vi "Agilent VNA Sort Measurements.vi"(7 "Agilent VNA":T6, 8 "error in (no error)":errorcluster, 9 "Auto Select":bool, 10 "Parameters to Measure":T1[](array[typedef]) {"Channel" min=1 max=99 step=1; "Parameter"."Stimulus Port" min=1 step=1; "Parameter"."Response Port" min=1 step=1}, 11 "VISA Resource Name":refnum<visa-resource-name>) -> (0 "error out":errorcluster {"code" format="%.0x"}, 1 "Channels Used":i8[](array[numeric]), 2 "Sorted Measurements":cluster{"Measurements":T5[]}[](array[cluster]) {"Measurements"."Traces"."Parameter"."Stimulus Port" min=1 step=1; "Measurements"."Traces"."Parameter"."Response Port" min=1 step=1}, 3 "dup VISA Resource Name":refnum<visa-resource-name>, 4 "Sorted Parameters to Measure":T1[](array[typedef]) {"Channel" min=1 max=99 step=1; "Parameter"."Stimulus Port" min=1 step=1; "Parameter"."Response Port" min=1 step=1}, 5 "Removed Parameters":T1[](array[typedef]) {"Channel" min=1 max=99 step=1; "Parameter"."Stimulus Port" min=1 step=1; "Parameter"."Response Port" min=1 step=1}, 6 "Measurements Removed?":bool)   [LabVIEW 2011]
uses:
  tests/S Parameter/TypeDefs/SP Parameter to Measure.ctl
  tests/S Parameter/TypeDefs/SP Parameter.ctl
  tests/S Parameter/TypeDefs/SP Calibration State.ctl
  tests/S Parameter/TypeDefs/SP Measurement Format.ctl
  TypeDefs/Agilent VNA Instrument Info.ctl
  TypeDefs/Agilent VNA Measurements.ctl
  SI.LIB/Add to Array if Not Present (I32).vi
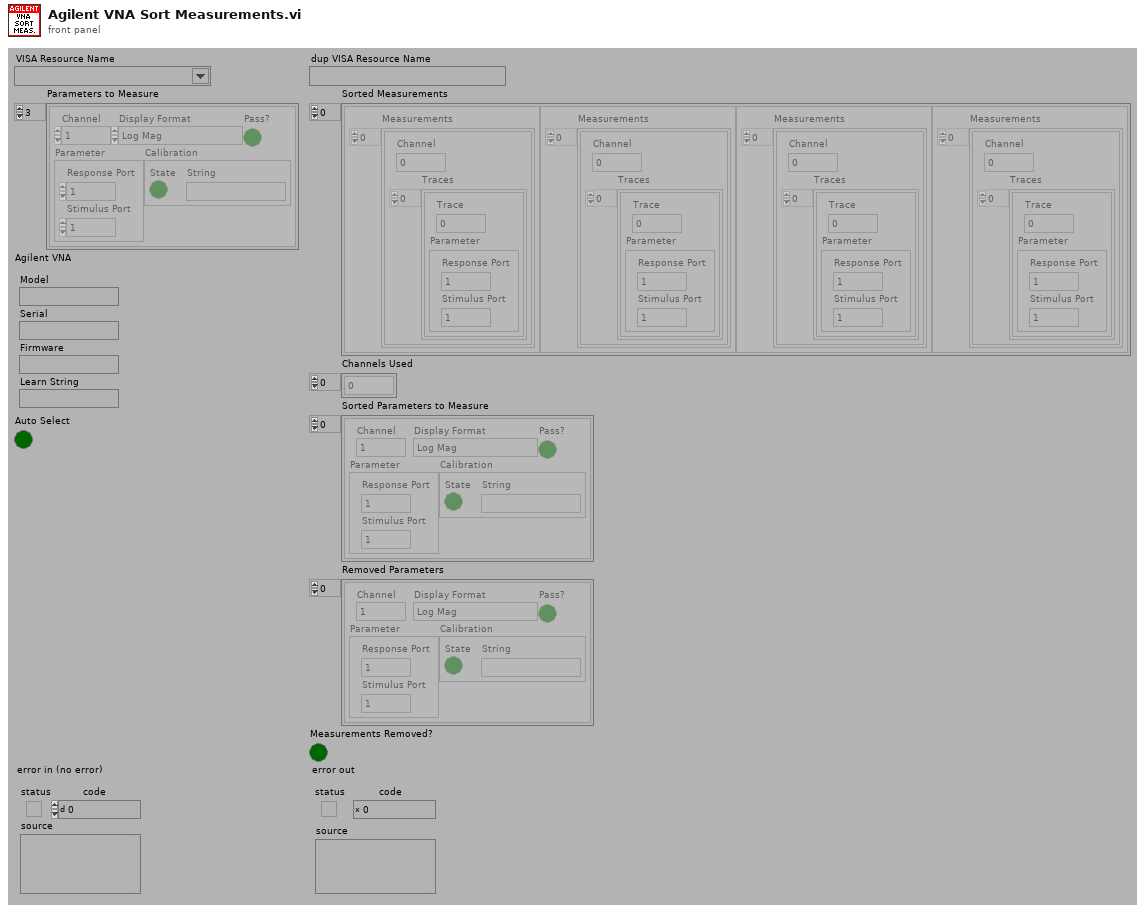
[diagram p1: front panel]
types:
  T1 = typedef "SP Parameter to Measure.ctl" = cluster{"Channel":i8, "Parameter":T2, "Calibration":T3, "Display Format":T4, "Pass?":bool}
  T2 = typedef "SP Parameter.ctl" = cluster{"Stimulus Port":i8, "Response Port":i8}
  T3 = typedef "SP Calibration State.ctl" = cluster{"State":bool, "String":string}
  T4 = typedef "SP Measurement Format.ctl" = enum32{"Log Mag", "Phase", "Delay", "Smith (R+jX)", "Polar (Re/Im)", "Linear Mag", "SWR", "Real", "Imaginary", "Smith (Lin/Phase)", "Smith (Log/Phase)", "Smith (Real/Imag)", "Smith (G+jB)", "Polar (Lin/Phase)", "Polar (Log/Phase)", "Expanded Phase", "Positive Phase", "Inverted Smith", "Unwrapped Phase", "Power Out", "Power In", "Linear Mag/Phase", "Log Mag/Phase", "Real/Imaginary"}
  T5 = typedef "Agilent VNA Measurements.ctl" = cluster{"Channel":i8, "Traces":cluster{"Trace":i8, "Parameter":T2}[]}
  T6 = typedef "Agilent VNA Instrument Info.ctl" = cluster{"Model":string, "Serial":string, "Firmware":string, "Learn String":string}
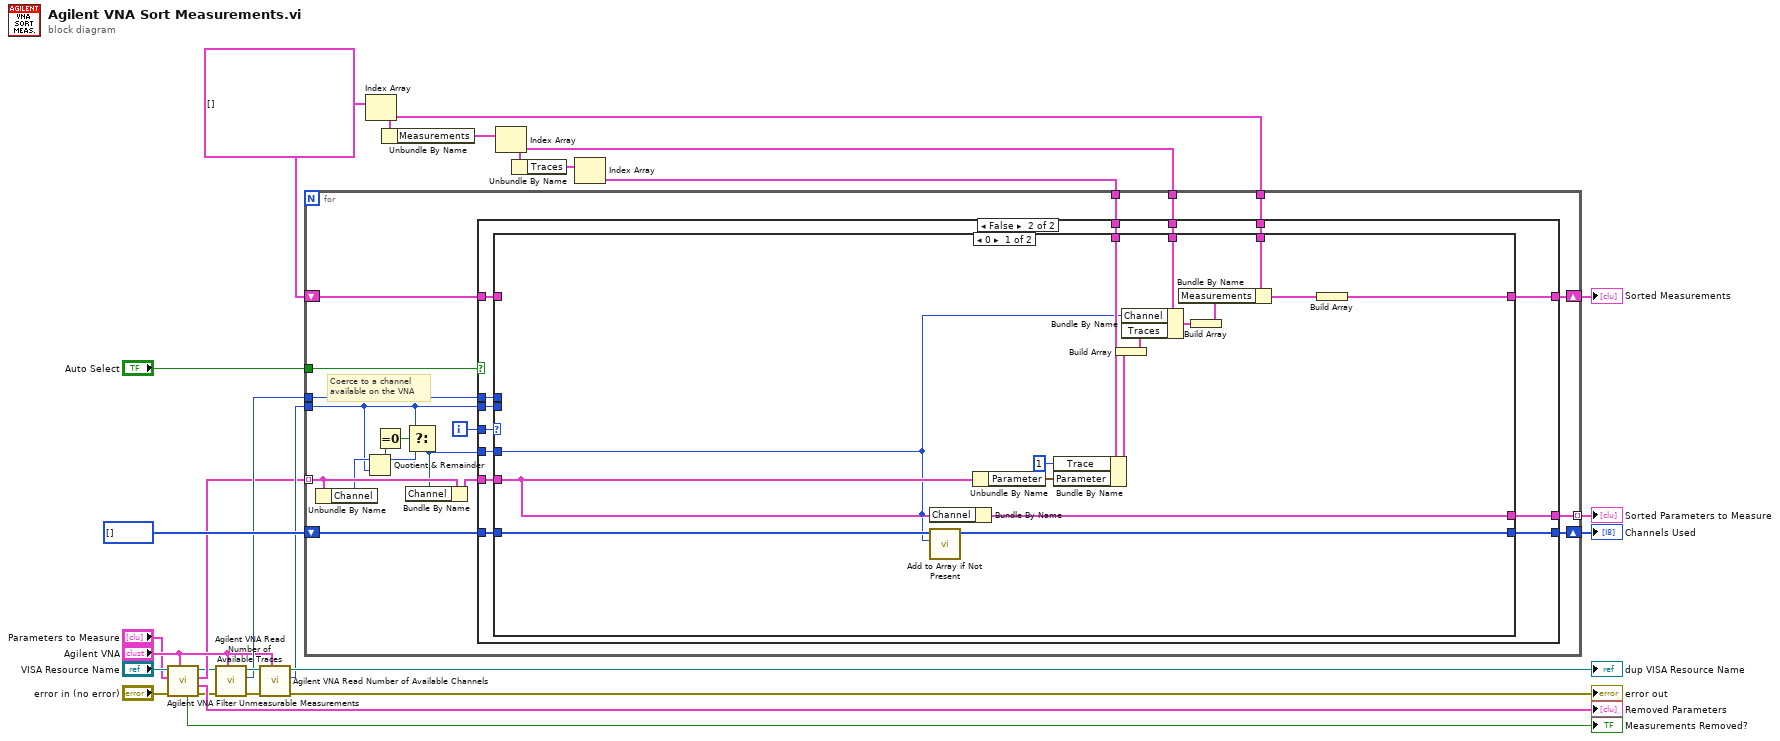
[diagram p0: block diagram]
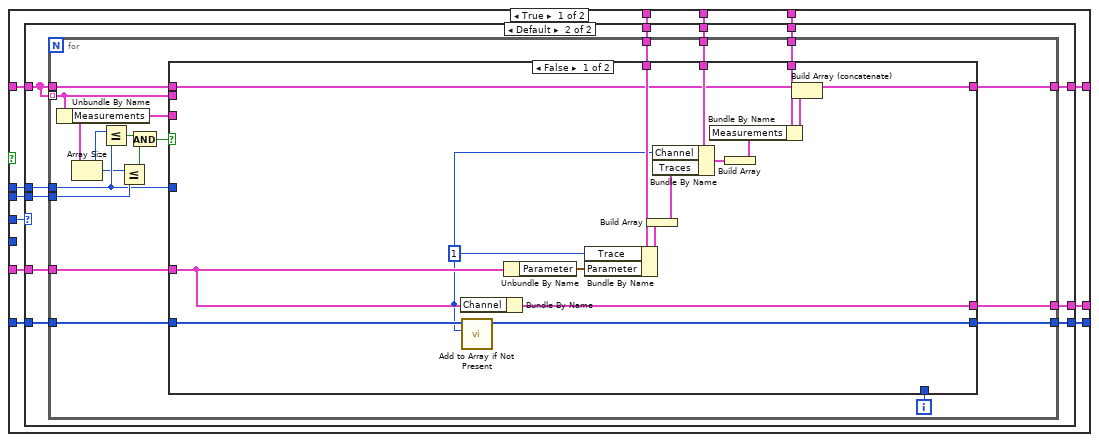
[diagram p2: hidden frame]
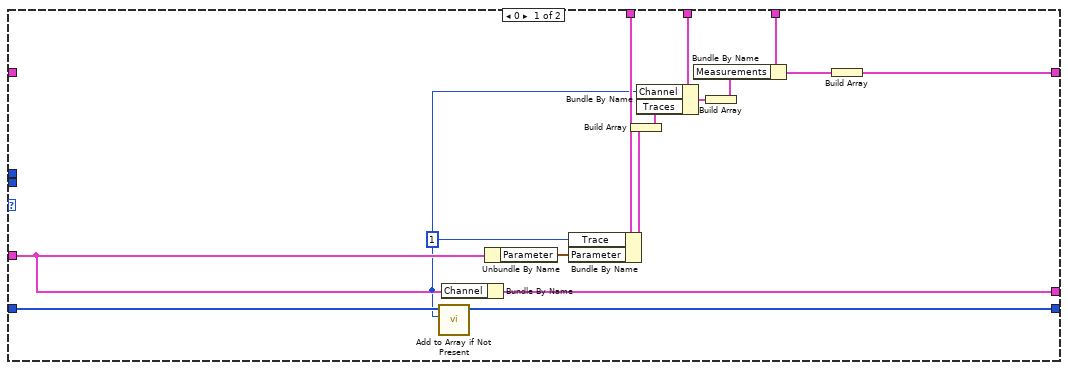
[diagram p3: hidden frame]
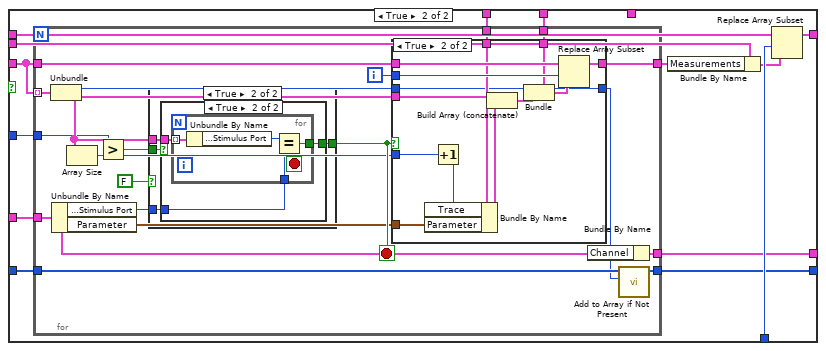
[diagram p4: hidden frame]
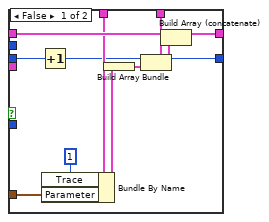
[diagram p7: hidden frame]
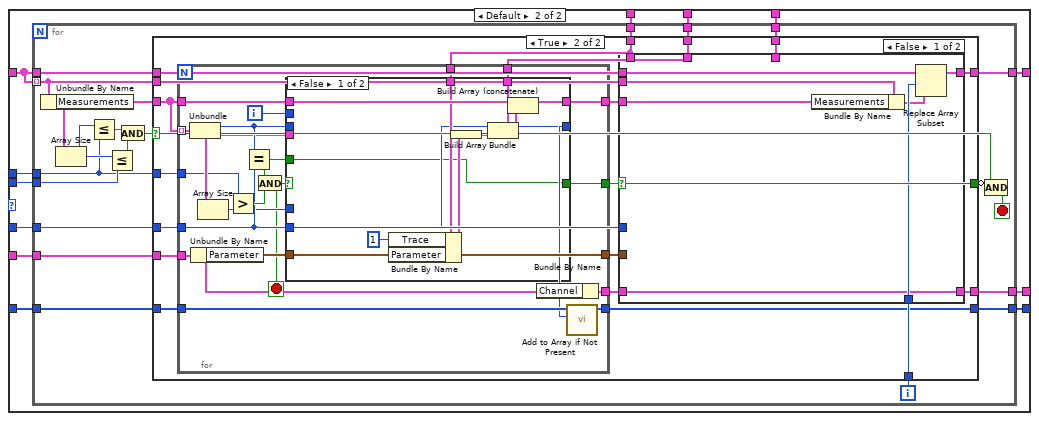
[diagram p8: hidden frame]
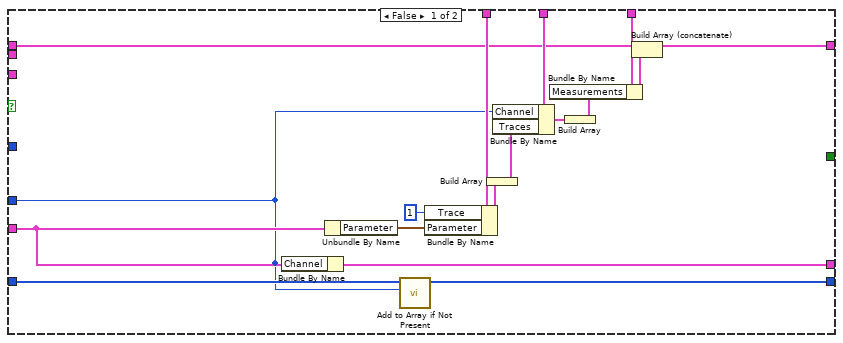
[diagram p9: hidden frame]
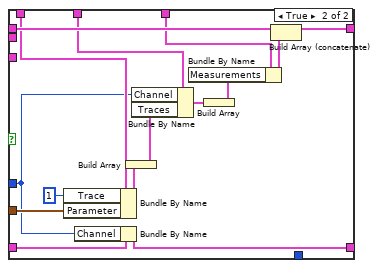
[diagram p10: hidden frame]
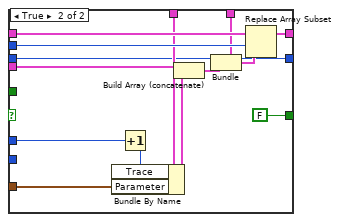
[diagram p11: hidden frame]
diagram:
  w21 = cluster{"Measurements":T5[]}[] [] ("Sorted Measurements")
  n1 = call "Agilent VNA Filter Unmeasurable Measurements.vi"("Agilent VNA"="Agilent VNA", "error in (no error)"="error in (no error)", "Parameters to Measure"="Parameters to Measure", "VISA Resource Name"="VISA Resource Name") -> ("error out"=w1:errorcluster, "Removed Parameters"=→"Removed Parameters":T1[], "Filtered Parameters to Measure"=w6:T1[], "dup VISA Resource Name"=w2:refnum<visa-resource-name>, "Measurements Removed?"=→"Measurements Removed?":bool)  [unwired: 3 out]
  n2 = call "Agilent VNA Read Number of Available Traces.vi"("Agilent VNA"="Agilent VNA", "error in (no error)"=w1, "VISA Resource Name"=w2) -> ("error out"=w13:errorcluster, "Number of Traces"=w11:i8, "dup VISA Resource Name"=w12:refnum<visa-resource-name>)  [unwired: 6 out]
  n3 = call "Agilent VNA Read Number of Available Channels.vi"("Agilent VNA"="Agilent VNA", "error in (no error)"=w13, "VISA Resource Name"=w12) -> ("error out"=→"error out":errorcluster, "Number of Channels"=w14:i8, "dup VISA Resource Name"=→"dup VISA Resource Name":refnum<visa-resource-name>)  [unwired: 6 out]
  n4 = Index Array(array=w21) -> (element=w17:cluster{"Measurements":T5[]})  [unwired: 1 in]
  n5 = Unbundle By Name(w17) -> ("Measurements"=w23:T5[])
  n6 = Index Array(array=w23) -> (element=w18:T5)  [unwired: 1 in]
  n7 = Unbundle By Name(w18) -> ("Traces"=w20:cluster{"Trace":i8, "Parameter":T2}[])
  n8 = Index Array(array=w20) -> (element=w19:cluster{"Trace":i8, "Parameter":T2})  [unwired: 1 in]
  n9 = for {
    tunnel: w6 -> [w42] mode=indexing
    shift-right: [w32] -> w22
    shift-left: w21 -> [w43]
    tunnel: w14 -> [w37]
    tunnel: "Auto Select" -> [w35]
    tunnel: w19 -> [w34]
    tunnel: w18 -> [w33]
    tunnel: w17 -> [w31]
    shift-right: [w29] -> w15
    shift-left: i8[] [] -> [w30]
    tunnel: w11 -> [w28]
    tunnel: [w27] -> w5 mode=indexing
    i -> [w44]
    # "Coerce to a channel\navailable on the VNA"
    n10 = Unbundle By Name(w42) -> ("Channel"=w40:i8)
    n11 = Quotient & Remainder(x=w40, y=w37) -> (x-y*floor(x/y)=w36:i8)  [unwired: 1 out]
    n12 = Equal To 0?(x=w36) -> (x = 0?=w39:bool)
    n13 = Select(t=w37, s=w39, f=w36) -> (s? t:f=w38:i8)
    n14 = Bundle By Name(cluster=w42, "Channel"=w38) -> (w41:T1)
    n15 = case shown="False" w35 {
      tunnel: w44 -> [w50 w194]
      tunnel: w43 -> [w56 w200]
      tunnel: w41 -> [w55 w199]
      tunnel: w38 -> [_ w190]
      tunnel: w37 -> [w54 w198]
      tunnel: w34 -> [w53 w197]
      tunnel: w33 -> [w52 w196]
      tunnel: [w51 w195] -> w32
      tunnel: w31 -> [w49 w193]
      tunnel: w30 -> [w48 w192]
      tunnel: [w47 w191] -> w29
      tunnel: w28 -> [w46 w189]
      tunnel: [w45 w188] -> w27
      frame True {
        n16 = case shown="Default" w50 {
          tunnel: w56 -> [_ w77]
          tunnel: w55 -> [w59 w82]
          tunnel: w54 -> [_ w81]
          tunnel: w53 -> [w71 w80]
          tunnel: w52 -> [w69 w79]
          tunnel: [w62 w78] -> w51
          tunnel: w49 -> [w65 w76]
          tunnel: w48 -> [w61 w75]
          tunnel: [w60 w74] -> w47
          tunnel: w46 -> [_ w73]
          tunnel: [w57 w72] -> w45
          frame 0 {
            w58 = i8 1 ("Trace")
            n17 = call-poly "Add to Array if Not Present.vi"("I32"=w58, "I32 Array"=w61) -> ("New I32 Array"=w60:i32[])  [unwired: 3 out]
            n18 = Bundle By Name(cluster=w59, "Channel"=w58) -> (w57:T1)
            n19 = Unbundle By Name(w59) -> ("Parameter"=w70:T2)
            n20 = Bundle By Name(cluster=w71, "Trace"=w58, "Parameter"=w70) -> (w67:cluster{"Trace":i8, "Parameter":T2})
            n21 = Build Array(w67) -> (w66:cluster{"Trace":i8, "Parameter":T2}[])
            n22 = Bundle By Name(cluster=w69, "Channel"=w58, "Traces"=w66) -> (w68:T5)
            n23 = Build Array(w68) -> (w64:T5[])
            n24 = Bundle By Name(cluster=w65, "Measurements"=w64) -> (w63:cluster{"Measurements":T5[]})
            n25 = Build Array(w63) -> (w62:cluster{"Measurements":T5[]}[])
          }
          frame Default {
            n26 = for {
              tunnel: w77 -> [w96]
              tunnel: w82 -> [w100]
              tunnel: w81 -> [w85]
              tunnel: w80 -> [w99]
              tunnel: w79 -> [w98]
              tunnel: [w97] -> w78
              tunnel: w77 -> [w92] mode=indexing
              tunnel: w76 -> [w93]
              tunnel: w75 -> [w91]
              tunnel: [w90] -> w74
              tunnel: w73 -> [w84]
              tunnel: [w89] -> w72
              i -> [w95]
              n27 = Unbundle By Name(w92) -> ("Measurements"=w94:T5[])
              n28 = Array Size(array=w94) -> (size(s)=w83:i32)
              n29 = Less Or Equal?(x=w83, y=w84) -> (x <= y?=w87:bool)
              n30 = Less Or Equal?(x=w83, y=w85) -> (x <= y?=w88:bool)
              n31 = And(x=w87, y=w88) -> (x .and. y?=w86:bool)
              n32 = case shown="False" w86 {
                tunnel: w100 -> [w103 w130]
                tunnel: w99 -> [w114 w129]
                tunnel: w98 -> [w113 w128]
                tunnel: [w116 w125] -> w97
                tunnel: w94 -> [_ w127]
                tunnel: w96 -> [w110 w126]
                tunnel: w95 -> [_ w124]
                tunnel: w93 -> [w108 _]
                tunnel: w92 -> [_ w123]
                tunnel: w91 -> [w105 w120]
                tunnel: [w104 w119] -> w90
                tunnel: w84 -> [_ w118]
                tunnel: [w102 w117] -> w89
                frame False {
                  w101 = i8 1 ("Channel")
                  n33 = Bundle By Name(cluster=w103, "Channel"=w101) -> (w102:T1)
                  n34 = call-poly "Add to Array if Not Present.vi"("I32"=w101, "I32 Array"=w105) -> ("New I32 Array"=w104:i32[])  [unwired: 3 out]
                  n35 = Unbundle By Name(w103) -> ("Parameter"=w115:T2)
                  n36 = Bundle By Name(cluster=w114, "Trace"=w101, "Parameter"=w115) -> (w112:cluster{"Trace":i8, "Parameter":T2})
                  n37 = Build Array(w112) -> (w111:cluster{"Trace":i8, "Parameter":T2}[])
                  n38 = Bundle By Name(cluster=w113, "Channel"=w101, "Traces"=w111) -> (w109:T5)
                  n39 = Build Array(w109) -> (w107:T5[])
                  n40 = Bundle By Name(cluster=w108, "Measurements"=w107) -> (w106:cluster{"Measurements":T5[]})
                  n41 = Build Array (concatenate)(w110, w106) -> (w116:cluster{"Measurements":T5[]}[])
                }
                frame True {
                  n42 = for {
                    tunnel: w127 -> [w146] mode=indexing
                    tunnel: w130 -> [w134]
                    tunnel: w127 -> [w150]
                    tunnel: [w147] -> w122
                    tunnel: w129 -> [w142]
                    tunnel: w128 -> [w140]
                    tunnel: w120 -> [w137]
                    tunnel: [w136] -> w119
                    tunnel: w118 -> [w135]
                    tunnel: [w133] -> w117
                    i -> [w149]
                    stop <- w145 stop-if-true
                    n43 = Unbundle(w146) -> ("Channel"=w143:i8, "Traces"=w144:cluster{"Trace":i8, "Parameter":T2}[])
                    n44 = Unbundle By Name(w134) -> ("Parameter.Stimulus Port"=w138:i8, "Parameter"=w139:T2)
                    n45 = Array Size(array=w144) -> (size(s)=w141:i32)
                    n46 = Greater?(x=w135, y=w141) -> (0:w148:bool)
                    n47 = case shown="True" FALSE {
                      tunnel: w148 -> [w151 w155]
                      tunnel: [w151 w154] -> w145
                      tunnel: w144 -> [_ w153]
                      tunnel: w138 -> [_ w152]
                      frame False {
                        # "We are no longer sorting by\nstimulus port.  We have decided\nthat it is no faster since it has to\nsweep once for each stimulus\nport no matter the configuration."
                      }
                      frame True {
                        n48 = case shown="True" w155 {
                          selector: w155 -> [w156 _]
                          tunnel: w153 -> [_ w159]
                          tunnel: [w156 w158] -> w154
                          tunnel: w152 -> [_ w157]
                          frame False {
                          }
                          frame True {
                            n49 = for {
                              tunnel: w159 -> [w163] mode=indexing
                              tunnel: [w161] -> w158
                              tunnel: w157 -> [w160]
                              stop <- w161 stop-if-true
                              n50 = Unbundle By Name(w163) -> ("Parameter.Stimulus Port"=w162:i8)
                              n51 = Equal?(x=w162, y=w160) -> (x = y?=w161:bool)
                            }
                          }
                        }
                      }
                    }
                    n52 = case shown="True" w145 {
                      tunnel: w144 -> [_ w183]
                      tunnel: w150 -> [w174 w187]
                      tunnel: w149 -> [_ w186]
                      tunnel: [w173 w185] -> w147
                      tunnel: w143 -> [w166 w175]
                      tunnel: w139 -> [w169 w181]
                      tunnel: w142 -> [w168 w182]
                      tunnel: w141 -> [_ w180]
                      tunnel: w140 -> [w170 w177]
                      tunnel: [w164 w175] -> w132
                      frame False {
                        n53 = Increment(x=w166) -> (x+1=w164:i8)
                        n54 = Bundle By Name(cluster=w168, "Trace"=i8 1, "Parameter"=w169) -> (w167:cluster{"Trace":i8, "Parameter":T2})
                        n55 = Build Array(w167) -> (w171:cluster{"Trace":i8, "Parameter":T2}[])
                        n56 = Bundle(cluster=w170, "Channel"=w164, "Traces"=w171) -> (w172:T5)
                        n57 = Build Array (concatenate)(w174, w172) -> (w173:T5[])
                      }
                      frame True {
                        n58 = Increment(x=w180) -> (x+1=w179:i32)
                        n59 = Bundle By Name(cluster=w182, "Trace"=w179, "Parameter"=w181) -> (w178:cluster{"Trace":i8, "Parameter":T2})
                        n60 = Build Array (concatenate)(w183, w178) -> (w176:cluster{"Trace":i8, "Parameter":T2}[])
                        n61 = Bundle(cluster=w177, "Channel"=w175, "Traces"=w176) -> (w184:T5)
                        n62 = Replace Array Subset(array=w187, new element=w184, index=w186) -> (w185:T5[])
                      }
                    }
                    n63 = Bundle By Name(cluster=w134, "Channel"=w132) -> (w133:T1)
                    n64 = call-poly "Add to Array if Not Present.vi"("I32"=w132, "I32 Array"=w137) -> ("New I32 Array"=w136:i32[])  [unwired: 3 out]
                  }
                  n65 = Bundle By Name(cluster=w123, "Measurements"=w122) -> (w121:cluster{"Measurements":T5[]})
                  n66 = Replace Array Subset(array=w126, new element=w121, index=w124) -> (w125:cluster{"Measurements":T5[]}[])
                }
              }
            }
          }
        }
      }
      frame False {
        n67 = case shown="0" w194 {
          tunnel: w200 -> [_ w223]
          tunnel: w199 -> [w204 w228]
          tunnel: w198 -> [_ w227]
          tunnel: w197 -> [w216 w226]
          tunnel: w196 -> [w214 w225]
          tunnel: [w207 w224] -> w195
          tunnel: w193 -> [w210 w222]
          tunnel: w192 -> [w206 w221]
          tunnel: [w205 w220] -> w191
          tunnel: w190 -> [w201 w219]
          tunnel: w189 -> [_ w218]
          tunnel: [w203 w217] -> w188
          frame 0 {
            n68 = Bundle By Name(cluster=w204, "Channel"=w201) -> (w203:T1)
            n69 = call-poly "Add to Array if Not Present.vi"("I32"=w201, "I32 Array"=w206) -> ("New I32 Array"=w205:i32[])  [unwired: 3 out]
            n70 = Unbundle By Name(w204) -> ("Parameter"=w215:T2)
            n71 = Bundle By Name(cluster=w216, "Trace"=i8 1 ("Channel"), "Parameter"=w215) -> (w212:cluster{"Trace":i8, "Parameter":T2})
            n72 = Build Array(w212) -> (w211:cluster{"Trace":i8, "Parameter":T2}[])
            n73 = Bundle By Name(cluster=w214, "Channel"=w201, "Traces"=w211) -> (w213:T5)
            n74 = Build Array(w213) -> (w209:T5[])
            n75 = Bundle By Name(cluster=w210, "Measurements"=w209) -> (w208:cluster{"Measurements":T5[]})
            n76 = Build Array(w208) -> (w207:cluster{"Measurements":T5[]}[])
          }
          frame Default {
            n77 = for {
              tunnel: w223 -> [w245]
              tunnel: w228 -> [w249]
              tunnel: w227 -> [w231]
              tunnel: w226 -> [w248]
              tunnel: w225 -> [w247]
              tunnel: [w246] -> w224
              tunnel: w223 -> [w242] mode=indexing
              tunnel: w222 -> [w243]
              tunnel: w221 -> [w241]
              tunnel: [w240] -> w220
              tunnel: w219 -> [w239]
              tunnel: w218 -> [w229]
              tunnel: [w236] -> w217
              i -> [w244]
              stop <- w237 stop-if-true
              n78 = Unbundle By Name(w242) -> ("Measurements"=w233:T5[])
              n79 = Array Size(array=w233) -> (size(s)=w230:i32)
              n80 = Less Or Equal?(x=w230, y=w229) -> (x <= y?=w234:bool)
              n81 = Less Or Equal?(x=w230, y=w231) -> (x <= y?=w235:bool)
              n82 = And(x=w234, y=w235) -> (x .and. y?=w232:bool)
              n83 = case shown="True" w232 {
                tunnel: w249 -> [w252 w284]
                tunnel: w248 -> [w264 w275]
                tunnel: w247 -> [w263 w274]
                tunnel: [w266 w281] -> w246
                tunnel: w233 -> [_ w283]
                tunnel: w245 -> [w260 w282]
                tunnel: w244 -> [_ w280]
                tunnel: w243 -> [w258 w271]
                tunnel: w242 -> [_ w279]
                tunnel: w241 -> [w255 w277]
                tunnel: [w254 w276] -> w240
                tunnel: w239 -> [w251 w272]
                tunnel: [_ w270] -> w238
                tunnel: w229 -> [_ w269]
                tunnel: [w250 w268] -> w236
                frame False {
                  n84 = Bundle By Name(cluster=w252, "Channel"=w251) -> (w250:T1)
                  n85 = Unbundle By Name(w252) -> ("Parameter"=w265:T2)
                  n86 = call-poly "Add to Array if Not Present.vi"("I32"=w251, "I32 Array"=w255) -> ("New I32 Array"=w254:i32[])  [unwired: 3 out]
                  n87 = Bundle By Name(cluster=w264, "Trace"=i8 1 ("Channel"), "Parameter"=w265) -> (w262:cluster{"Trace":i8, "Parameter":T2})
                  n88 = Build Array(w262) -> (w261:cluster{"Trace":i8, "Parameter":T2}[])
                  n89 = Bundle By Name(cluster=w263, "Channel"=w251, "Traces"=w261) -> (w259:T5)
                  n90 = Build Array(w259) -> (w257:T5[])
                  n91 = Bundle By Name(cluster=w258, "Measurements"=w257) -> (w256:cluster{"Measurements":T5[]})
                  n92 = Build Array (concatenate)(w260, w256) -> (w266:cluster{"Measurements":T5[]}[])
                }
                frame True {
                  n93 = for {
                    tunnel: w283 -> [w324] mode=indexing
                    tunnel: w284 -> [w309]
                    tunnel: w283 -> [w327]
                    tunnel: [w325] -> w278
                    tunnel: w275 -> [w323]
                    tunnel: w274 -> [w322]
                    tunnel: w277 -> [w321]
                    tunnel: [w320] -> w276
                    tunnel: w272 -> [w315]
                    tunnel: [w318] -> w273
                    tunnel: [w312] -> w270
                    tunnel: w269 -> [w310]
                    tunnel: [w307] -> w267
                    i -> [w326]
                    stop <- w313 stop-if-true
                    n94 = Unbundle(w324) -> ("Channel"=w319:i8, "Traces"=w317:cluster{"Trace":i8, "Parameter":T2}[])
                    n95 = Unbundle By Name(w309) -> ("Parameter"=w318:T2)
                    n96 = Array Size(array=w317) -> (size(s)=w314:i32)
                    n97 = Greater?(x=w310, y=w314) -> (0:w316:bool)
                    n98 = Equal?(x=w319, y=w315) -> (x = y?=w311:bool)
                    n99 = And(x=w311, y=w316) -> (x .and. y?=w313:bool)
                    n100 = case shown="False" w313 {
                      tunnel: w317 -> [_ w348]
                      tunnel: w327 -> [w338 w352]
                      tunnel: w326 -> [_ w351]
                      tunnel: [w337 w350] -> w325
                      tunnel: w319 -> [_ w342]
                      tunnel: w318 -> [w331 w346]
                      tunnel: w323 -> [w333 w347]
                      tunnel: w322 -> [w334 w344]
                      tunnel: [w329 w342] -> w308
                      tunnel: w315 -> [w329 _]
                      tunnel: w314 -> [_ w341]
                      tunnel: [w328 FALSE] -> w312
                      tunnel: w311 -> [w328 _]
                      frame False {
                        n101 = Bundle By Name(cluster=w333, "Trace"=i8 1, "Parameter"=w331) -> (w332:cluster{"Trace":i8, "Parameter":T2})
                        n102 = Build Array(w332) -> (w335:cluster{"Trace":i8, "Parameter":T2}[])
                        n103 = Bundle(cluster=w334, "Channel"=w329, "Traces"=w335) -> (w336:T5)
                        n104 = Build Array (concatenate)(w338, w336) -> (w337:T5[])
                      }
                      frame True {
                        n105 = Increment(x=w341) -> (x+1=w340:i32)
                        n106 = Bundle By Name(cluster=w347, "Trace"=w340, "Parameter"=w346) -> (w345:cluster{"Trace":i8, "Parameter":T2})
                        n107 = Build Array (concatenate)(w348, w345) -> (w343:cluster{"Trace":i8, "Parameter":T2}[])
                        n108 = Bundle(cluster=w344, "Channel"=w342, "Traces"=w343) -> (w349:T5)
                        n109 = Replace Array Subset(array=w352, new element=w349, index=w351) -> (w350:T5[])
                      }
                    }
                    n110 = Bundle By Name(cluster=w309, "Channel"=w308) -> (w307:T1)
                    n111 = call-poly "Add to Array if Not Present.vi"("I32"=w308, "I32 Array"=w321) -> ("New I32 Array"=w320:i32[])  [unwired: 3 out]
                  }
                  n112 = case shown="False" w270 {
                    tunnel: w282 -> [w291 w300]
                    tunnel: [w290 w299] -> w281
                    tunnel: w280 -> [w289 _]
                    tunnel: w279 -> [w288 _]
                    tunnel: w278 -> [w287 _]
                    tunnel: w275 -> [_ w298]
                    tunnel: w274 -> [_ w296]
                    tunnel: w273 -> [_ w297]
                    tunnel: w272 -> [_ w292]
                    tunnel: w271 -> [_ w295]
                    tunnel: [w285 w293] -> w268
                    tunnel: w267 -> [w285 w294]
                    frame False {
                      n113 = Bundle By Name(cluster=w288, "Measurements"=w287) -> (w286:cluster{"Measurements":T5[]})
                      n114 = Replace Array Subset(array=w291, new element=w286, index=w289) -> (w290:cluster{"Measurements":T5[]}[])
                    }
                    frame True {
                      n115 = Bundle By Name(cluster=w298, "Trace"=i8 1 ("Channel"), "Parameter"=w297) -> (w306:cluster{"Trace":i8, "Parameter":T2})
                      n116 = Bundle By Name(cluster=w294, "Channel"=w292) -> (w293:T1)
                      n117 = Build Array(w306) -> (w305:cluster{"Trace":i8, "Parameter":T2}[])
                      n118 = Bundle By Name(cluster=w296, "Channel"=w292, "Traces"=w305) -> (w304:T5)
                      n119 = Build Array(w304) -> (w303:T5[])
                      n120 = Bundle By Name(cluster=w295, "Measurements"=w303) -> (w302:cluster{"Measurements":T5[]})
                      n121 = Build Array (concatenate)(w300, w302) -> (w299:cluster{"Measurements":T5[]}[])
                    }
                  }
                }
              }
              n122 = Compound Arithmetic op=AND(invert w238, w232) -> (w237:bool)
            }
          }
        }
      }
    }
  }
  "Sorted Measurements" <- w22
  "Channels Used" <- w15
  "Sorted Parameters to Measure" <- w5
